vi "Robot Arm Portcullis.vi"(8 "Motor Speed":dbl, 9 "Limit Switch Shoulder":bool, 10 "Limit Switch Elbow":bool, 11 "Start Portcullis":bool) -> (0 "Done":bool, 1 "Arcade Drive":cluster{"x":dbl, "y":dbl}, 2 "Set Elbow":dbl, 3 "Set Shoulder":dbl)   [LabVIEW 2015]
uses:
  portcullis_auto_states.ctl
  Sensors.vi
panel:
  in  "Kd":dbl=0.005
  in  "Kp":dbl=0.05
  in  "Ki":dbl
  in  "Drive Time":dbl
  in  "Abort":bool
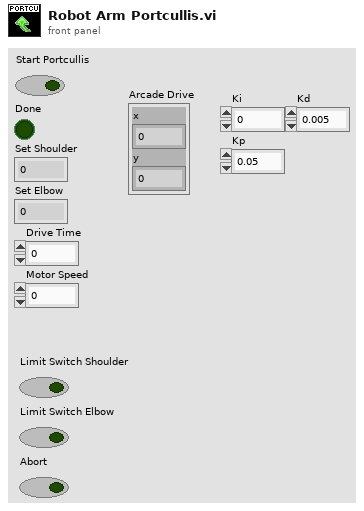
[diagram p1: front panel]
types:
  T1 = typedef "portcullis_auto_states.ctl" = enum16{"Ready", "Arm to Gate", "Drive to Gate", "Arm Hook In", "Arm up", "Drive Thru", "Move to rest", "Stop"}
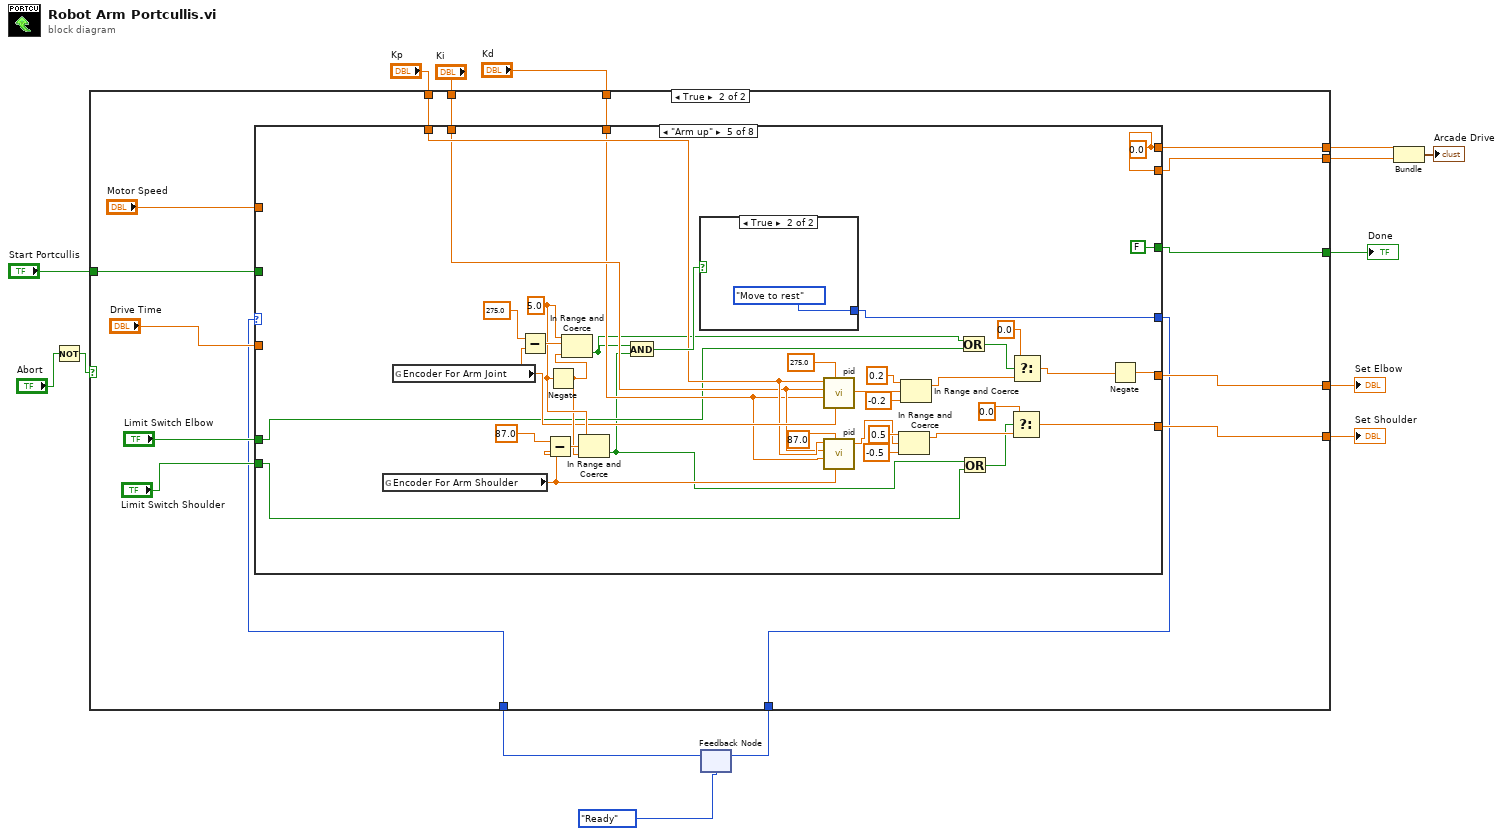
[diagram p0: block diagram]
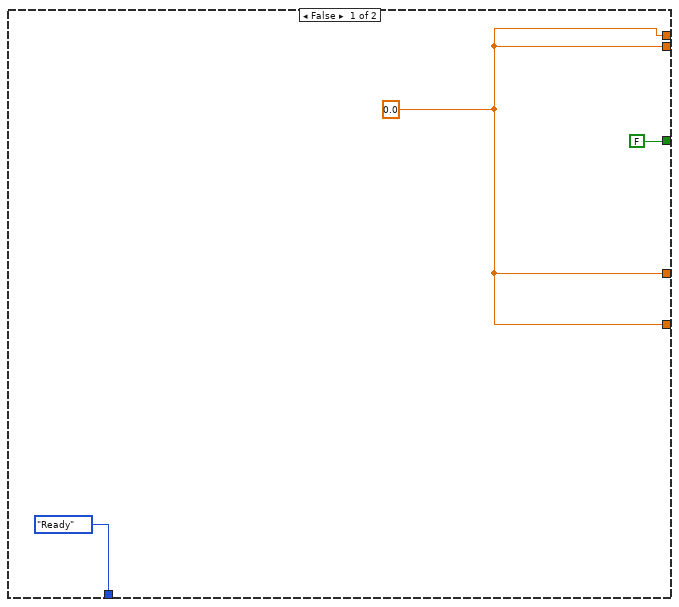
[diagram p2: hidden frame]
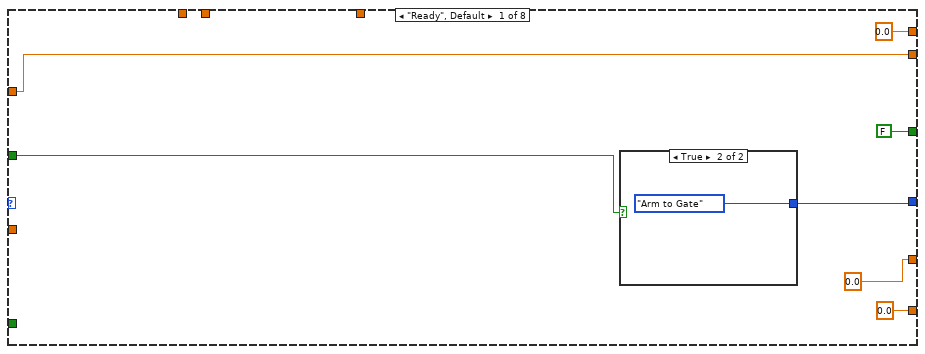
[diagram p3: hidden frame]
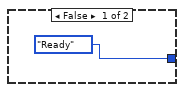
[diagram p4: hidden frame]
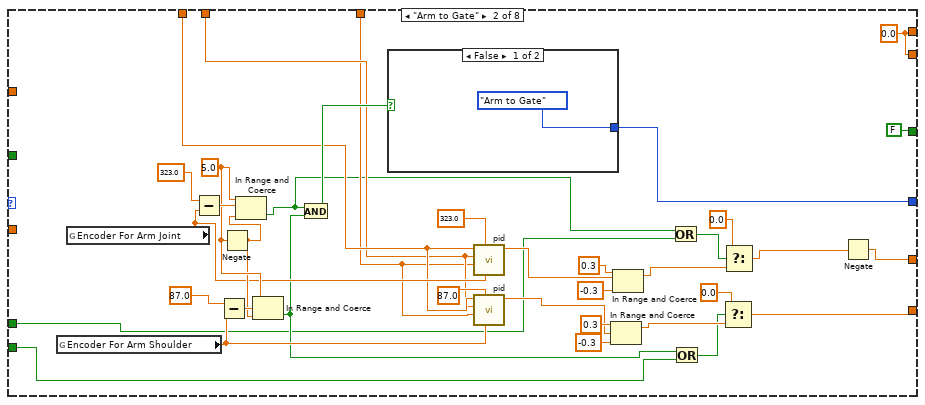
[diagram p5: hidden frame]
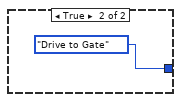
[diagram p6: hidden frame]
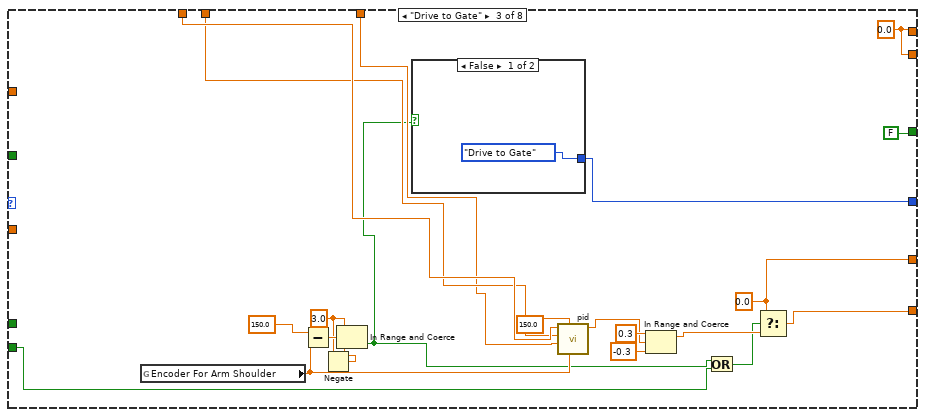
[diagram p7: hidden frame]
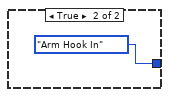
[diagram p8: hidden frame]
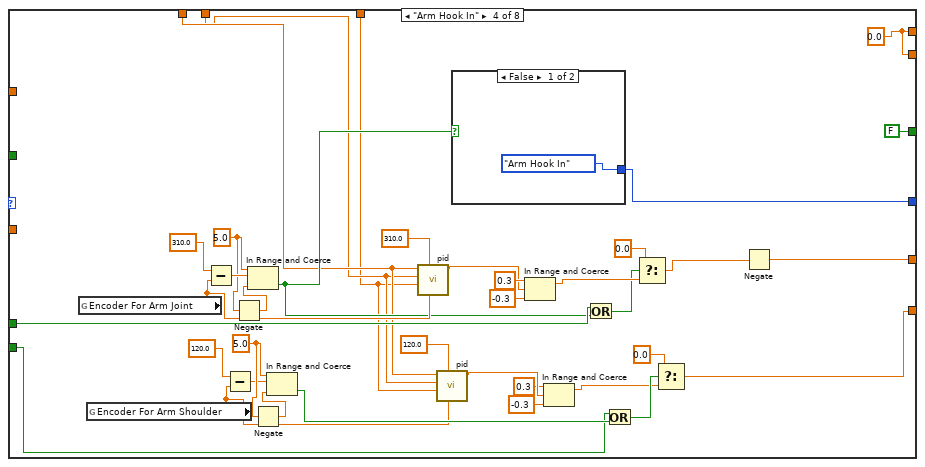
[diagram p9: hidden frame]
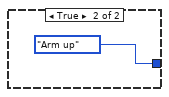
[diagram p10: hidden frame]
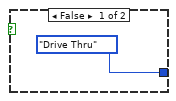
[diagram p11: hidden frame]
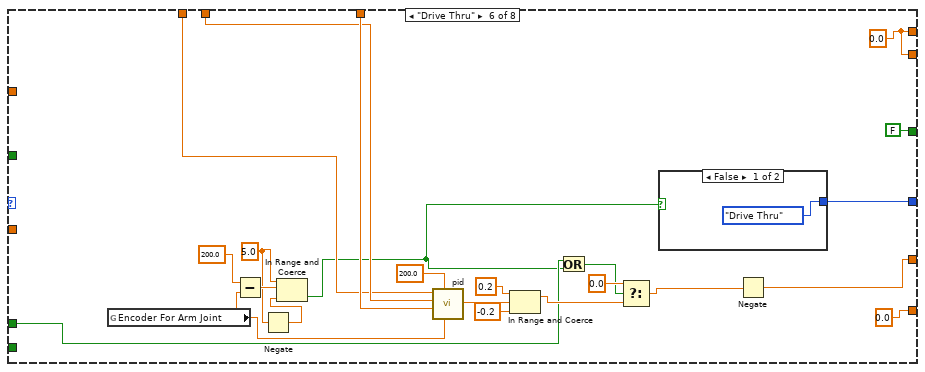
[diagram p12: hidden frame]
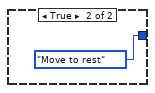
[diagram p13: hidden frame]
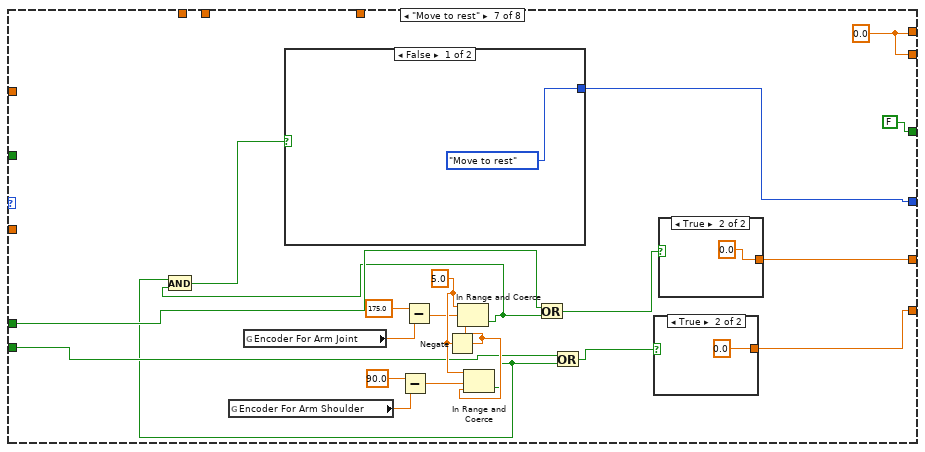
[diagram p14: hidden frame]
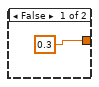
[diagram p15: hidden frame]
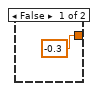
[diagram p16: hidden frame]
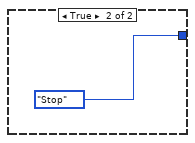
[diagram p17: hidden frame]
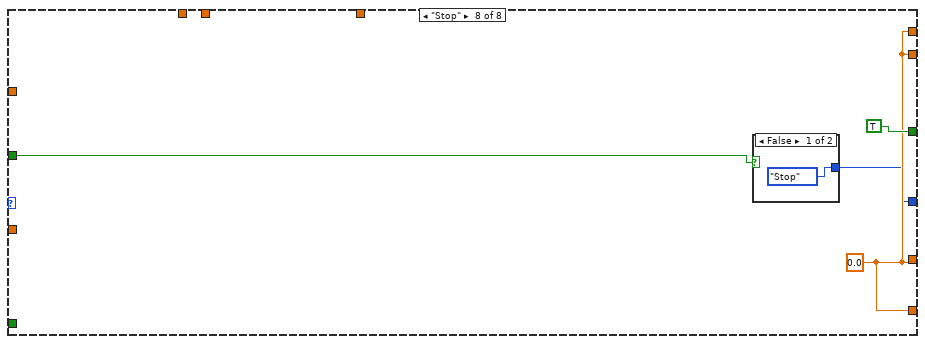
[diagram p18: hidden frame]
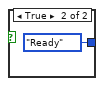
[diagram p19: hidden frame]
diagram:
  n1 = Not(x="Abort") -> (.not. x?=w9:bool)
  n2 = feedback #1(portcullis_auto_states."Ready") -> (w2:T1)
  n3 = case shown="True" w9 {
    tunnel: [w18 w29] -> w15
    tunnel: [w18 w28] -> w14
    tunnel: [FALSE w27] -> w13
    tunnel: [w18 w26] -> w12
    tunnel: [w18 w25] -> w11
    tunnel: "Start Portcullis" -> [_ w24]
    tunnel: "Kd" -> [_ w23]
    tunnel: "Ki" -> [_ w22]
    tunnel: "Kp" -> [_ w21]
    tunnel: w2 -> [_ w20]
    tunnel: [portcullis_auto_states."Ready" w19] -> w1
    frame False {
      w18 = 0.0
    }
    frame True {
      n4 = case shown="\"Arm up\"" w20 {
        tunnel: "Motor Speed" -> [w40 _ _ _ _ _ _ _]
        tunnel: "Drive Time" -> [_ _ _ _ _ _ _ _]
        tunnel: [0.0 w66 w81 w140 w143 w182 w224 w234] -> w29
        tunnel: [FALSE FALSE FALSE FALSE FALSE FALSE FALSE TRUE] -> w27
        tunnel: [0.0 ("Set Motor at S") w50 w85 w122 w151 w189 w221 w234] -> w26
        tunnel: [0.0 ("Set Motor at 1") w47 w87 w104 w144 0.0 w222 w234] -> w25
        tunnel: [w40 w66 w81 w140 w143 w182 w224 w234] -> w28
        tunnel: "Limit Switch Shoulder" -> [_ w43 w86 w105 w145 _ w210 _]
        tunnel: "Limit Switch Elbow" -> [_ w44 _ w125 w148 w184 w211 _]
        tunnel: [w35 w65 w100 w138 w167 w203 w220 w233] -> w19
        tunnel: w24 -> [w34 _ _ _ _ _ _ w232]
        tunnel: w23 -> [_ w62 w93 w106 w164 w193 _ _]
        tunnel: w22 -> [_ w63 w94 w107 w165 w192 _ _]
        tunnel: w21 -> [_ w64 w95 w108 w166 w191 _ _]
        frame "Ready", Default {
          n5 = case shown="True" w34 {
            tunnel: [portcullis_auto_states."Ready" portcullis_auto_states."Arm to Gate"] -> w35
            frame False {
            }
            frame True {
            }
          }
        }
        frame "Arm to Gate" {
          w70 = 5.0
          w66 = 0.0
          n6 = global read "Sensors.vi" "Encoder For Arm Shoulder"() -> (w68:dbl)
          n7 = global read "Sensors.vi" "Encoder For Arm Joint"() -> (w67:dbl)
          n8 = Subtract(x=323.0 ("setpoint"), y=w67) -> (x-y=w72:dbl)
          n9 = Subtract(x=87.0 ("setpoint"), y=w68) -> (x-y=w75:dbl)
          n10 = Negate(x=w70) -> (-x=w69:dbl)
          n11 = In Range and Coerce(upper limit=w70, x=w72, lower limit=w69) -> (In Range?=w46:bool)  [unwired: 1 out]
          n12 = In Range and Coerce(upper limit=w70, x=w75, lower limit=w69) -> (In Range?=w45:bool)  [unwired: 1 out]
          n13 = And(x=w46, y=w45) -> (x .and. y?=w73:bool)
          n14 = case shown="False" w73 {
            tunnel: [portcullis_auto_states."Arm to Gate" portcullis_auto_states."Drive to Gate"] -> w65
            frame False {
            }
            frame True {
            }
          }
          n15 = call "pid.vi"("y"=w67, "setpoint"=323.0, "kd"=w62, "ki"=w63, "kp"=w64) -> ("Motor Command"=w49:dbl)  [unwired: 6 in]
          n16 = call "pid.vi"("y"=w68, "setpoint"=87.0, "kd"=w62, "ki"=w63, "kp"=w64) -> ("Motor Command"=w48:dbl)  [unwired: 6 in]
          n17 = In Range and Coerce(upper limit=0.3, x=w48, lower limit=-0.3) -> (coerced(x)=w60:dbl)  [unwired: 1 out]
          n18 = In Range and Coerce(upper limit=0.3, x=w49, lower limit=-0.3) -> (coerced(x)=w61:dbl)  [unwired: 1 out]
          n19 = Or(x=w46, y=w44) -> (x .or. y?=w56:bool)
          n20 = Or(x=w45, y=w43) -> (x .or. y?=w57:bool)
          n21 = Select(t=0.0, s=w57, f=w60) -> (s? t:f=w47:dbl)
          n22 = Select(t=0.0, s=w56, f=w61) -> (s? t:f=w51:dbl)
          n23 = Negate(x=w51) -> (-x=w50:dbl)
        }
        frame "Drive to Gate" {
          w84 = 3.0 ("upper limit")
          w85 = 0.0
          w81 = 0.0
          n24 = global read "Sensors.vi" "Encoder For Arm Shoulder"() -> (w96:dbl)
          n25 = Subtract(x=150.0 ("setpoint"), y=w96) -> (x-y=w98:dbl)
          n26 = Negate(x=w84) -> (-x=w83:dbl)
          n27 = In Range and Coerce(upper limit=w84, x=w98, lower limit=w83) -> (In Range?=w82:bool)  [unwired: 1 out]
          n28 = case shown="False" w82 {
            tunnel: [portcullis_auto_states."Drive to Gate" portcullis_auto_states."Arm Hook In"] -> w100
            frame False {
            }
            frame True {
            }
          }
          n29 = call "pid.vi"("y"=w96, "setpoint"=150.0, "kd"=w93, "ki"=w94, "kp"=w95) -> ("Motor Command"=w88:dbl)  [unwired: 6 in]
          n30 = In Range and Coerce(upper limit=0.3, x=w88, lower limit=-0.3) -> (coerced(x)=w92:dbl)  [unwired: 1 out]
          n31 = Or(x=w82, y=w86) -> (x .or. y?=w91:bool)
          n32 = Select(t=w85, s=w91, f=w92) -> (s? t:f=w87:dbl)
        }
        frame "Arm Hook In" {
          w111 = 5.0
          w135 = 5.0
          w140 = 0.0
          n33 = global read "Sensors.vi" "Encoder For Arm Joint"() -> (w133:dbl)
          n34 = global read "Sensors.vi" "Encoder For Arm Shoulder"() -> (w113:dbl)
          n35 = Subtract(x=310.0 ("setpoint"), y=w133) -> (x-y=w137:dbl)
          n36 = Subtract(x=120.0 ("setpoint"), y=w113) -> (x-y=w109:dbl)
          n37 = Negate(x=w135) -> (-x=w134:dbl)
          n38 = In Range and Coerce(upper limit=w135, x=w137, lower limit=w134) -> (In Range?=w124:bool)  [unwired: 1 out]
          n39 = Negate(x=w111) -> (-x=w112:dbl)
          n40 = In Range and Coerce(upper limit=w111, x=w109, lower limit=w112) -> (In Range?=w121:bool)  [unwired: 1 out]
          n41 = call "pid.vi"("y"=w133, "setpoint"=310.0, "kd"=w106, "ki"=w107, "kp"=w108) -> ("Motor Command"=w126:dbl)  [unwired: 6 in]
          n42 = call "pid.vi"("y"=w113, "setpoint"=120.0, "kd"=w106, "ki"=w107, "kp"=w108) -> ("Motor Command"=w120:dbl)  [unwired: 6 in]
          n43 = case shown="False" w124 {
            tunnel: [portcullis_auto_states."Arm Hook In" portcullis_auto_states."Arm up"] -> w138
            frame False {
            }
            frame True {
            }
          }
          n44 = In Range and Coerce(upper limit=0.3, x=w126, lower limit=-0.3) -> (coerced(x)=w131:dbl)  [unwired: 1 out]
          n45 = In Range and Coerce(upper limit=0.3, x=w120, lower limit=-0.3) -> (coerced(x)=w115:dbl)  [unwired: 1 out]
          n46 = Or(x=w125, y=w124) -> (x .or. y?=w130:bool)
          n47 = Or(x=w105, y=w121) -> (x .or. y?=w116:bool)
          n48 = Select(t=0.0, s=w130, f=w131) -> (s? t:f=w123:dbl)
          n49 = Select(t=0.0, s=w116, f=w115) -> (s? t:f=w104:dbl)
          n50 = Negate(x=w123) -> (-x=w122:dbl)
        }
        frame "Arm up" {
          w173 = 5.0
          w143 = 0.0
          n51 = global read "Sensors.vi" "Encoder For Arm Shoulder"() -> (w163:dbl)
          n52 = global read "Sensors.vi" "Encoder For Arm Joint"() -> (w169:dbl)
          n53 = Subtract(x=275.0 ("setpoint"), y=w169) -> (x-y=w175:dbl)
          n54 = Subtract(x=87.0 ("setpoint"), y=w163) -> (x-y=w177:dbl)
          n55 = Negate(x=w173) -> (-x=w172:dbl)
          n56 = In Range and Coerce(upper limit=w173, x=w175, lower limit=w172) -> (In Range?=w147:bool)  [unwired: 1 out]
          n57 = In Range and Coerce(upper limit=w173, x=w177, lower limit=w172) -> (In Range?=w146:bool)  [unwired: 1 out]
          n58 = And(x=w147, y=w146) -> (x .and. y?=w168:bool)
          n59 = case shown="True" w168 {
            tunnel: [portcullis_auto_states."Drive Thru" portcullis_auto_states."Move to rest"] -> w167
            frame False {
            }
            frame True {
            }
          }
          n60 = call "pid.vi"("y"=w169, "setpoint"=275.0, "kd"=w164, "ki"=w165, "kp"=w166) -> ("Motor Command"=w150:dbl)  [unwired: 6 in]
          n61 = call "pid.vi"("y"=w163, "setpoint"=87.0, "kd"=w164, "ki"=w165, "kp"=w166) -> ("Motor Command"=w149:dbl)  [unwired: 6 in]
          n62 = In Range and Coerce(upper limit=0.5, x=w149, lower limit=-0.5) -> (coerced(x)=w161:dbl)  [unwired: 1 out]
          n63 = In Range and Coerce(upper limit=0.2, x=w150, lower limit=-0.2) -> (coerced(x)=w162:dbl)  [unwired: 1 out]
          n64 = Or(x=w147, y=w148) -> (x .or. y?=w157:bool)
          n65 = Or(x=w146, y=w145) -> (x .or. y?=w158:bool)
          n66 = Select(t=0.0, s=w158, f=w161) -> (s? t:f=w144:dbl)
          n67 = Select(t=0.0, s=w157, f=w162) -> (s? t:f=w152:dbl)
          n68 = Negate(x=w152) -> (-x=w151:dbl)
        }
        frame "Drive Thru" {
          w182 = 0.0
          w199 = 5.0
          n69 = global read "Sensors.vi" "Encoder For Arm Joint"() -> (w190:dbl)
          n70 = Subtract(x=200.0 ("setpoint"), y=w190) -> (x-y=w201:dbl)
          n71 = Negate(x=w199) -> (-x=w198:dbl)
          n72 = In Range and Coerce(upper limit=w199, x=w201, lower limit=w198) -> (In Range?=w181:bool)  [unwired: 1 out]
          n73 = call "pid.vi"("y"=w190, "setpoint"=200.0, "kd"=w193, "ki"=w192, "kp"=w191) -> ("Motor Command"=w194:dbl)  [unwired: 6 in]
          n74 = In Range and Coerce(upper limit=0.2, x=w194, lower limit=-0.2) -> (coerced(x)=w187:dbl)  [unwired: 1 out]
          n75 = Or(x=w184, y=w181) -> (x .or. y?=w185:bool)
          n76 = Select(t=0.0, s=w185, f=w187) -> (s? t:f=w183:dbl)
          n77 = case shown="False" w181 {
            tunnel: [portcullis_auto_states."Drive Thru" portcullis_auto_states."Move to rest"] -> w203
            frame False {
            }
            frame True {
            }
          }
          n78 = Negate(x=w183) -> (-x=w189:dbl)
        }
        frame "Move to rest" {
          w219 = 5.0
          w224 = 0.0
          n79 = global read "Sensors.vi" "Encoder For Arm Shoulder"() -> (w215:dbl)
          n80 = global read "Sensors.vi" "Encoder For Arm Joint"() -> (w214:dbl)
          n81 = Subtract(x=90.0, y=w215) -> (x-y=w218:dbl)
          n82 = Subtract(x=175.0, y=w214) -> (x-y=w217:dbl)
          n83 = Negate(x=w219) -> (-x=w212:dbl)
          n84 = In Range and Coerce(upper limit=w219, x=w217, lower limit=w212) -> (In Range?=w207:bool)  [unwired: 1 out]
          n85 = In Range and Coerce(upper limit=w219, x=w218, lower limit=w212) -> (In Range?=w206:bool)  [unwired: 1 out]
          n86 = And(x=w206, y=w207) -> (x .and. y?=w223:bool)
          n87 = case shown="False" w223 {
            tunnel: [portcullis_auto_states."Move to rest" portcullis_auto_states."Stop"] -> w220
            frame False {
            }
            frame True {
            }
          }
          n88 = Or(x=w211, y=w207) -> (x .or. y?=w208:bool)
          n89 = Or(x=w210, y=w206) -> (x .or. y?=w209:bool)
          n90 = case shown="True" w209 {
            tunnel: [-0.3 0.0] -> w222
            frame False {
            }
            frame True {
            }
          }
          n91 = case shown="True" w208 {
            tunnel: [0.3 0.0] -> w221
            frame False {
            }
            frame True {
            }
          }
        }
        frame "Stop" {
          w234 = 0.0
          n92 = case shown="False" w232 {
            tunnel: [portcullis_auto_states."Stop" portcullis_auto_states."Ready"] -> w233
            frame False {
            }
            frame True {
            }
          }
        }
      }
    }
  }
  "Done" <- w13
  "Set Elbow" <- w12
  "Set Shoulder" <- w11
  n93 = feedback-in #1(w1) -> ()
  n94 = Bundle(w15, "Motor Speed"=w14) -> (→"Arcade Drive":cluster{dbl, "Motor Speed":dbl})  [unwired: 1 in]
